vi "GraphFormattingUSB.vi"(4 "Error In":errorcluster, 5 "GraphIndex":T1, 7 "dataIN":waveform(dbl)[](array[waveform]) caption="données") -> (0 "Error Out":errorcluster, 2 "Graph2Data":waveform(dbl)[](array[waveform]), 3 "Graph1Data":waveform(dbl)[](array[waveform]))   [LabVIEW 2017]
panel:
  out "taille(s)":i32
  out "Grph2Data":waveform(dbl)[][](array[waveform])
  out "Grph1Data":waveform(dbl)[][](array[waveform])
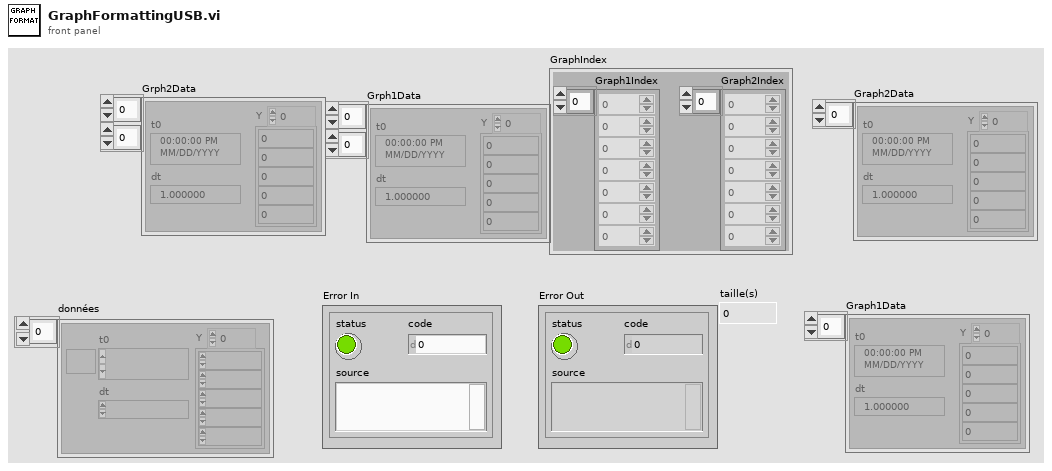
[diagram p1: front panel]
types:
  T1 = cluster{"Graph2Index":i32[], "Graph1Index":i32[]}
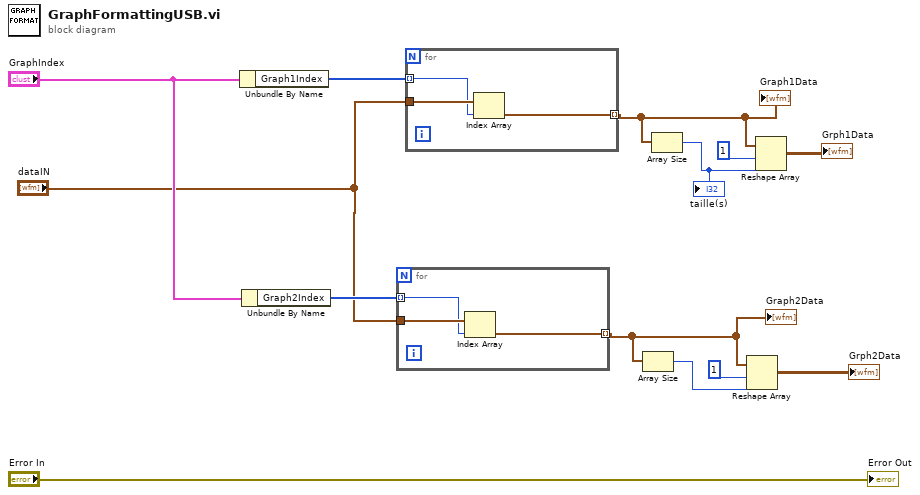
[diagram p0: block diagram]
diagram:
  n1 = Unbundle By Name("GraphIndex") -> ("Graph1Index"=w13:i32[])
  n2 = Unbundle By Name("GraphIndex") -> ("Graph2Index"=w5:i32[])
  n3 = for {
    tunnel: w5 -> [w15] mode=indexing
    tunnel: "dataIN" -> [w16]
    tunnel: [w14] -> w8 mode=indexing
    n4 = Index Array(array=w16, index=w15) -> (element=w14:waveform(dbl))
  }
  "Graph2Data" <- w8
  n5 = for {
    tunnel: w13 -> [w18] mode=indexing
    tunnel: "dataIN" -> [w19]
    tunnel: [w17] -> w10 mode=indexing
    n6 = Index Array(array=w19, index=w18) -> (element=w17:waveform(dbl))
  }
  "Graph1Data" <- w10
  n7 = Array Size(array=w8) -> (size(s)=w7:i32)
  n8 = Array Size(array=w10) -> (size(s)=w11:i32)
  "taille(s)" <- w11
  n9 = Reshape Array(w8, 1 ("taille de la dimension"), w7) -> (→"Grph2Data":waveform(dbl)[][])
  n10 = Reshape Array(w10, 1 ("taille de la dimension"), w11) -> (→"Grph1Data":waveform(dbl)[][])
  "Error Out" <- "Error In"
